vi "Stop Core.vi"(10 "final error code":i32, 11 "uService Template in":refnum<class "Kasli Wrapper 2.0.lvclass">) -> (3 "uService Template out":refnum<class "Kasli Wrapper 2.0.lvclass">)   [LabVIEW 2020, in "Kasli Wrapper 2.0.lvlib" / "Kasli Wrapper 2.0.lvclass"]
doc: "(<B>Filename</B>: Actor Framework.lvlib:Actor.lvclass:Stop Core.vi)\n\nDefines what the actor does before it stops. Use the <B>final error code</B> input to determine whether the actor shut down in response to an error.\n\nBy default, this method passes the Stop message along to all auto-stop nested actors. A descendant class may override this method to define additional behavior, such as shutting down any processes the actor initiated in its override of the Actor Core method."
uses:
  Kasli Wrapper 2.0.lvclass
  <vilib>/event_ctls.llb/usereventprio.ctl
  TALOS/TALOS_PPL.lvlibp
  Libraries/JKI_dotNET_System_Exec_PPL.lvlibp/dotnet_system_exec.lvclass
  TALOS/TALOS_PPL.lvlibp/Father of all uServices/Father of all uServices/Father of all uServices.lvclass
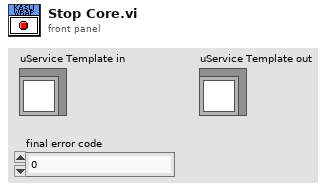
[diagram p1: front panel]
types:
  T1 = typedef "usereventprio.ctl" = enum32{"high priority", "normal priority"}
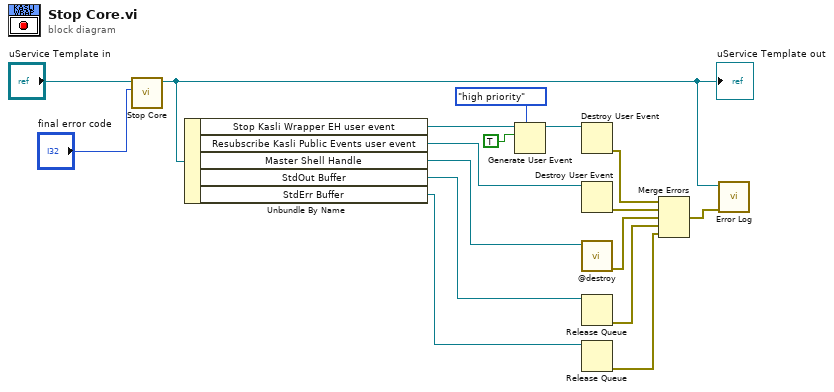
[diagram p0: block diagram]
diagram:
  n1 = call-parent "Stop Core.vi"("final error code"="final error code", "uService Template in"="uService Template in") -> ("uService Template out"=w8:refnum<class "Kasli Wrapper 2.0.lvclass">)  [unwired: 9 in]
  "uService Template out" <- w8
  n2 = Unbundle By Name(w8) -> ("Stop Kasli Wrapper EH user event"=w15:refnum<user-event>, "Resubscribe Kasli Public Events user event"=w11:refnum<user-event>, "Master Shell Handle"=w1:refnum<class "dotnet_system_exec.lvclass">, "StdOut Buffer"=w6:refnum<queue>, "StdErr Buffer"=w5:refnum<queue>)
  n3 = Generate User Event(priority (normal)=usereventprio."high priority", user event=w15, event data cluster=TRUE ("event data")) -> (user event out=w13:refnum<user-event>)  [unwired: 1 in, 1 out]
  n4 = Destroy User Event(user event=w13) -> (error out=w10:errorcluster)  [unwired: 1 in]
  n5 = Destroy User Event(user event=w11) -> (error out=w9:errorcluster)  [unwired: 1 in]
  n6 = call-dynamic "@destroy.vi"("dotnet_system_exec in"=w1) -> ("error out"=w2:errorcluster)  [unwired: 9 in, 1 out]
  n7 = Release Queue(queue=w6) -> (error out=w4:errorcluster)  [unwired: 2 in, 2 out]
  n8 = Release Queue(queue=w5) -> (error out=w3:errorcluster)  [unwired: 2 in, 2 out]
  n9 = Merge Errors(w10, w9, w2, w4, w3) -> (w7:errorcluster)
  n10 = call "Error Log.vi"("error in (no error)"=w7, "Object in"=w8) -> ()  [unwired: 9 in, 1 out]
